vi "数字波形的显示.vi"() -> ()   [LabVIEW 2010]
panel:
  out "数字数据":digitaldata
  out "数字波形图 2":digitalwaveform(graph)
  in  "16位整型数十进制格式":i16[](array[numeric])=[0, 13, 18, 26, 98, 30, 255]
  out "数字波形图":digitalwaveform(graph)
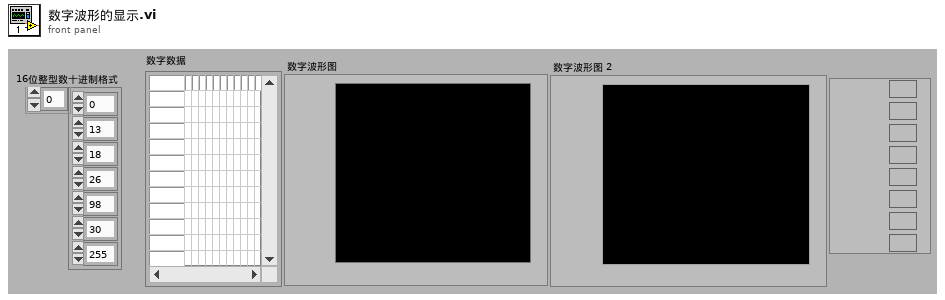
[diagram p1: front panel]
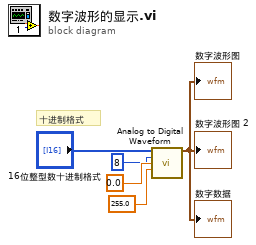
[diagram p0: block diagram]
diagram:
  # "十进制格式"
  n1 = call <vilib>:"Analog to Digital Waveform.vi"("Analog Waveform"="16位整型数十进制格式", "Resolution (16 bit)"=8, "Min (-1.0)"=0.0, "Max (1.0)"=255.0) -> ("Digital Waveform"=→"数字波形图" →"数字波形图 2" →"数字数据":digitalwaveform)  [unwired: 7 in, 4 out]
